vi "0036-Sub_GPIO_AllOff.vi"(8 "エラー出力 2":errorcluster caption="エラー入力", 11 "device":i32) -> (0 "エラー出力":errorcluster, 3 "deviceOut":T1)   [LabVIEW 2014]
uses:
  LVProject/private/CP2112_device.ctl
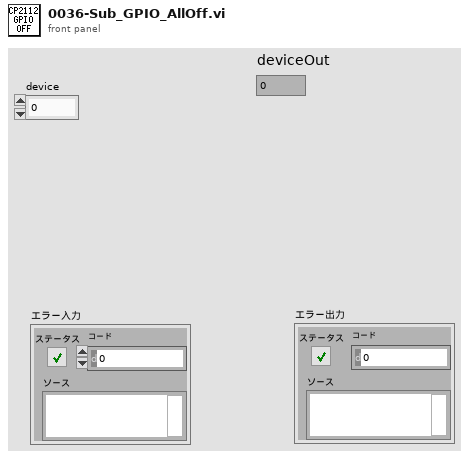
[diagram p1: front panel]
types:
  T1 = typedef "CP2112_device.ctl" = i32
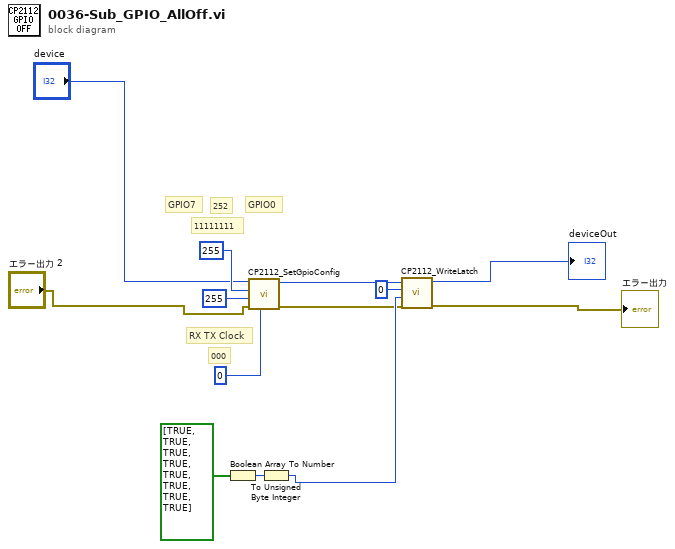
[diagram p0: block diagram]
diagram:
  # "252"
  # "RX TX Clock"
  # "GPIO7"
  # "GPIO0"
  # "000"
  # "11111111"
  n1 = Boolean Array To Number(Boolean array=bool[] [TRUE, TRUE, TRUE, TRUE, TRUE, TRUE, TRUE, TRUE] ("ブール配列")) -> (number=w2:u32)
  n2 = call "CP2112_SetGpioConfig.vi"("special"=u8 0, "error in (no error)"="エラー出力 2", "mode"=u8 255, "direction"=u8 255, "device"="device") -> ("error out"=w10:errorcluster, "deviceOut"=w11:T1)  [unwired: 4 in, 1 out]
  n3 = To Unsigned Byte Integer(number=w2) -> (unsigned 8bit integer=w13:u8)
  n4 = call "CP2112_WriteLatch.vi"("error in (no error)"=w10, "latchMask"=w13, "latchValue"=u8 0, "device"=w11) -> ("error out"=→"エラー出力":errorcluster, "deviceOut"=→"deviceOut":T1)  [unwired: 5 in, 1 out]
